vi "Simple Test Executive Test.vi"() -> ()   [LabVIEW 2017]
uses:
  <vilib>/gpm_packages/@cs/test-executive/Source/Test Executive/Executioner/Executioner.lvclass
  <vilib>/gpm_packages/@cs/persistence/source/XML/XML.lvclass
  C:/Program Files/National Instruments/LabVIEW 2017/vi.lib/gpm_packages/@cs/persistence/source/IPersist/IPersist.lvclass
  <vilib>/gpm_packages/@cs/test-executive/Source/Test Executive/TestExecutive/Test Executive.lvclass
  C:/Program Files/National Instruments/LabVIEW 2017/vi.lib/gpm_packages/@cs/test-executive/Source/Test Executive/ITestExecutive/ITest Executive.lvclass
  <vilib>/gpm_packages/@cs/run-time-assertions/Source/Assert Equal/Assert Equal.lvclass
  C:/Program Files/National Instruments/LabVIEW 2017/vi.lib/gpm_packages/@cs/run-time-assertions/Source/Assert/Assert.lvclass
  866dfd19-2fef-4b99-8a4a-1d31d88e504e.vi
  55b154ae-6d03-47ed-abc2-d28db7feda01.vi
  cb4faef1-3dab-41b9-9dd5-aad0424c17a6.vi
  bfcbba5b-45c6-4320-969f-3e3d3b66b4de.vi
  8564ab31-dd3a-4968-8861-3b4339f4920d.vi
  9b79477b-4d99-41b4-a2fb-9df7ea8afb31.vi
  6decda23-fb0c-4e77-ad71-e1f71655b843.vi
  71592cda-0d0e-4ea7-b138-086424aed341.vi
  0583369c-d912-4d49-be3f-0b23069dcf00.vi
  bffa5b7c-ecbc-40cd-a0d5-f9da2a76cf50.vi
  c9edba23-499d-4d6b-bf99-6c37c6a75b36.vi
  b25967a6-4fd7-4e76-b6fa-60230ccf68d8.vi
  5610abd5-5b24-4367-9a8b-cdb86ef1c489.vi
  b0752a74-c361-4210-a9fb-4ae4d881d9e9.vi
  8d04dc0f-32ed-4eef-804d-f0fb33ecb275.vi
  <vilib>/Utility/error.llb/Clear Errors.vi
  <vilib>/Utility/error.llb/Error Cluster From Error Code.vi
  <vilib>/gpm_packages/@cs/test-executive/Source/Test Executive/ITestExecutive/ITest Executive.lvclass
  <vilib>/gpm_packages/@cs/test-executive/Source/Test Executive/TestExecutive Ref/TestExecutive Ref.lvclass
panel:
  out "Attributes":i32[](array[numeric])
  out "Names":string[](array[string])
  out "Unique ID out":string
  out "Array":string[](array[string])
  out "Class":string
  out "Tag":i32
  out "Name":string
  out "Attribute 2":i32
  out "x = y?":bool
  out "variant":variant
  out "Attribute":variant
  out "class name":string
  in  "stop":bool
  out "error out":errorcluster
  in  "Loaded Test Exec":string(tree)
  out "Pointer?":bool
  in  "File Name":string
  in  "Folder":path
  in  "Saved Test Exec":string(tree)
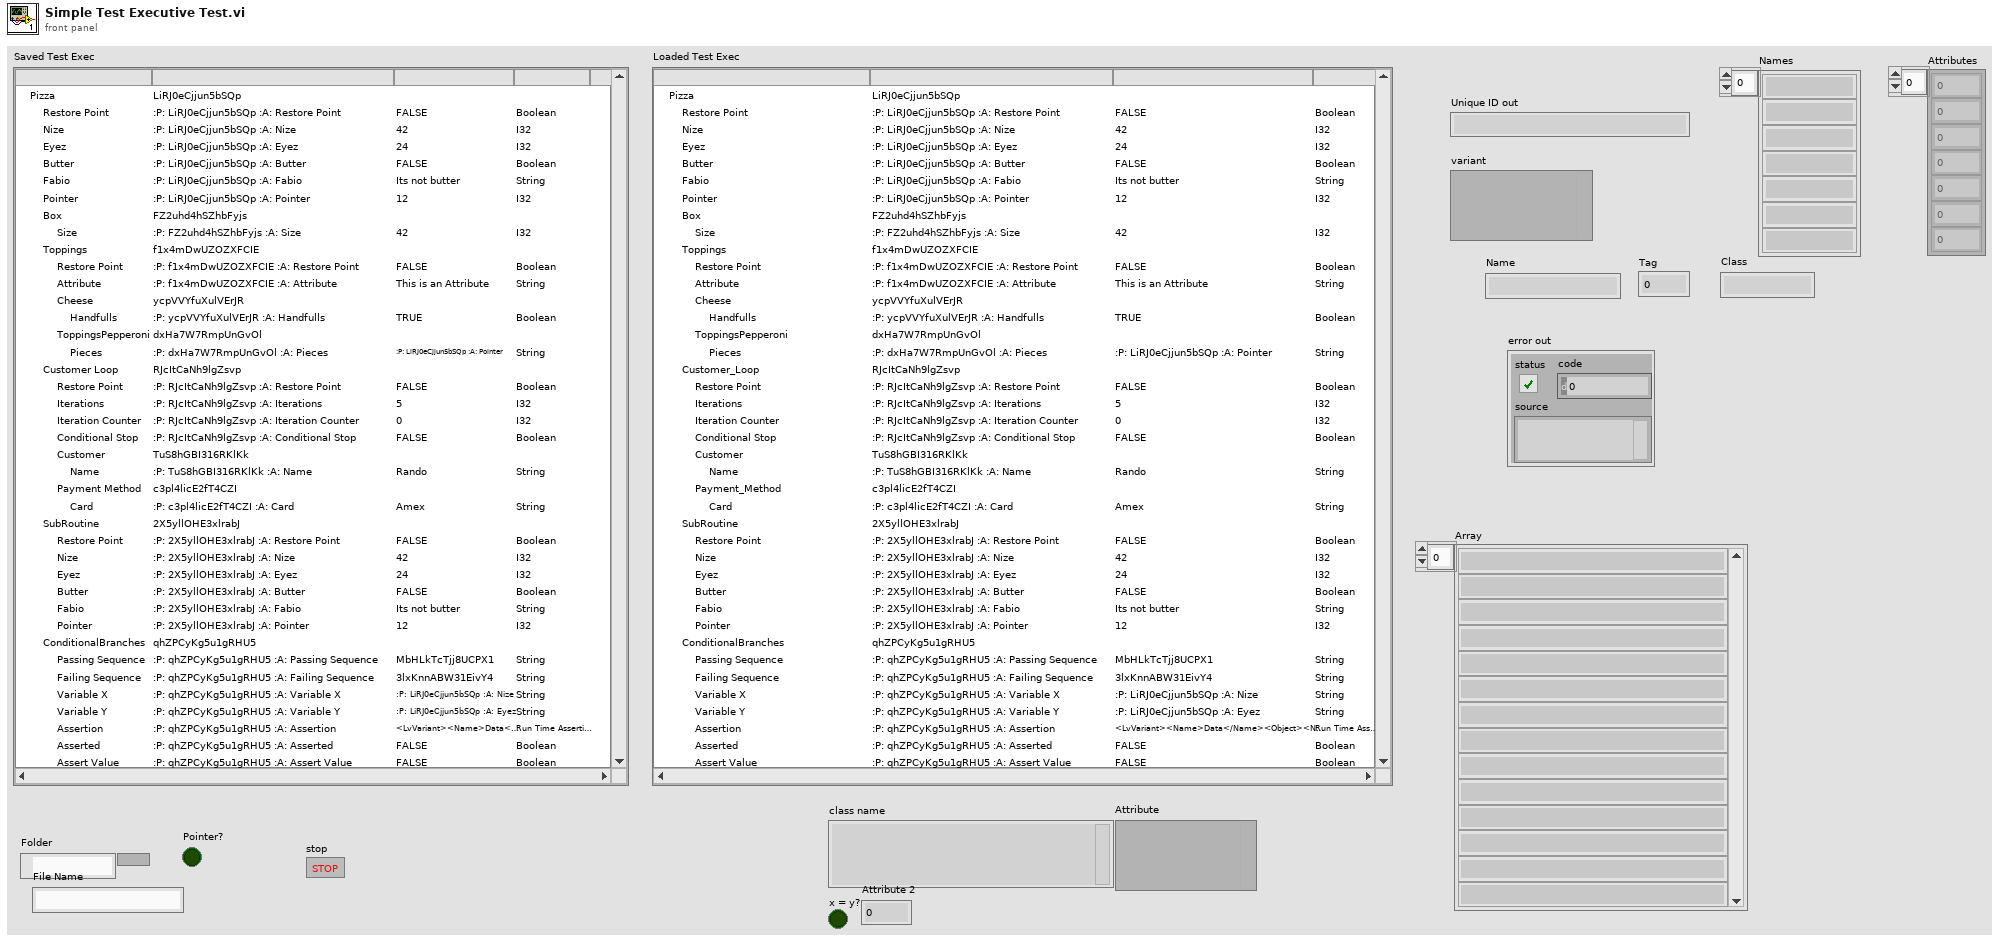
[diagram p1: front panel]
types:
  T1 = cluster{"Left Cell String":string, "Child Text":string[], "Child Tag":string, "Item Indent":i32, "Child Only?":bool, "Glyph Index":i32}[]
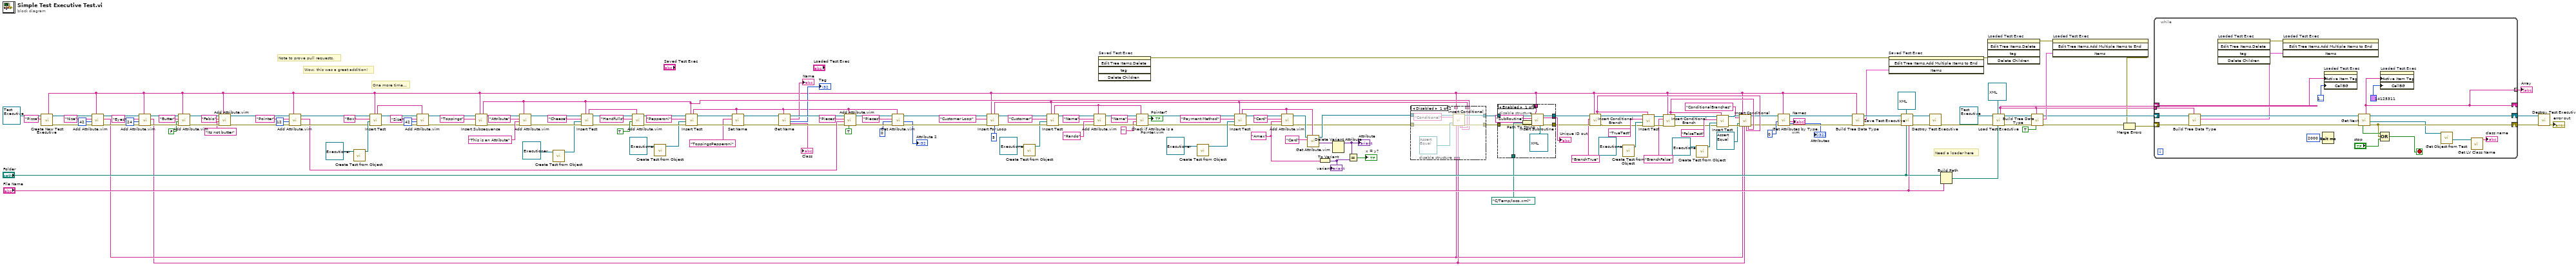
[diagram p0: block diagram]
diagram:
  w105 = "Amex"
  # "One more time..."
  # "Wow, this was a great addition!"
  # "Note to prove pull requests."
  # "Need a loader here"
  n1 = call <vilib>:"Create New Test Executive.vi"("Name"="Pizza", "Test Executive"=refnum<class "Test Executive.lvclass"> refnum ("Test Executive.lvlib:Test Executive.lvclass")) -> ("error out"=w99:errorcluster, "Test Executive Ref"=w100:refnum<data-value>, "Test Executive ID out"=w3:string)  [unwired: 7 in]
  n2 = call "Add Attribute.vim"("ID"=w3, "error in (no error)"=w99, "Attribute"=42, "Attribute Name"="Nize", "Test Executive Ref"=w100) -> ("error out"=w95:errorcluster, "Attribute ID out"=w5:string, "Test Executive Ref out"=w96:refnum<data-value>)  [unwired: 3 in, 1 out]
  n3 = call "Add Attribute.vim"("ID"=w3, "error in (no error)"=w95, "Attribute"=24, "Attribute Name"="Eyez", "Test Executive Ref"=w96) -> ("error out"=w36:errorcluster, "Attribute ID out"=w4:string, "Test Executive Ref out"=w37:refnum<data-value>)  [unwired: 3 in, 1 out]
  n4 = call "Add Attribute.vim"("ID"=w3, "error in (no error)"=w36, "Attribute"=FALSE, "Attribute Name"="Butter", "Test Executive Ref"=w37) -> ("error out"=w31:errorcluster, "Test Executive Ref out"=w33:refnum<data-value>)  [unwired: 3 in, 2 out]
  n5 = call "Add Attribute.vim"("ID"=w3, "error in (no error)"=w31, "Attribute"="Its not butter", "Attribute Name"="Fabio", "Test Executive Ref"=w33) -> ("error out"=w30:errorcluster, "Test Executive Ref out"=w32:refnum<data-value>)  [unwired: 3 in, 2 out]
  n6 = call "Add Attribute.vim"("ID"=w3, "error in (no error)"=w30, "Attribute"=12, "Attribute Name"="Pointer", "Test Executive Ref"=w32) -> ("error out"=w84:errorcluster, "Attribute ID out"=w82:string, "Test Executive Ref out"=w83:refnum<data-value>)  [unwired: 3 in, 1 out]
  n7 = call <vilib>:"Create Test from Object.vi"("Test"=refnum<class "Executioner.lvclass"> refnum ("Test Executive.lvlib:Executioner.lvclass")) -> ("Test"=w117:refnum<class "Executioner.lvclass">)  [unwired: 10 in]
  n8 = call <vilib>:"Insert Test.vi"("Parent ID"=w3, "error in (no error)"=w84, "Test"=w117, "Name"="Box", "Test Executive Ref"=w83) -> ("error out"=w141:errorcluster, "Test Executive Ref out"=w173:refnum<data-value>, "Unique ID out"=w172:string)  [unwired: 3 in, 1 out]
  n9 = call "Add Attribute.vim"("ID"=w172, "error in (no error)"=w141, "Attribute"=42, "Attribute Name"="Size", "Test Executive Ref"=w173) -> ("error out"=w91:errorcluster, "Test Executive Ref out"=w92:refnum<data-value>)  [unwired: 3 in, 2 out]
  n10 = call <vilib>:"Insert Subsequence.vi"("Parent ID"=w3, "error in (no error)"=w91, "Name"="Toppings", "Test Executive Ref"=w92) -> ("error out"=w140:errorcluster, "Test Executive Ref out"=w153:refnum<data-value>, "Unique ID out"=w87:string)  [unwired: 4 in, 1 out]
  n11 = call "Add Attribute.vim"("ID"=w87, "error in (no error)"=w140, "Attribute"="This is an Attribute", "Attribute Name"="Attribute", "Test Executive Ref"=w153) -> ("error out"=w139:errorcluster, "Test Executive Ref out"=w152:refnum<data-value>)  [unwired: 3 in, 2 out]
  n12 = call <vilib>:"Create Test from Object.vi"("Test"=refnum<class "Executioner.lvclass"> refnum ("Test Executive.lvlib:Executioner.lvclass")) -> ("Test"=w119:refnum<class "Executioner.lvclass">)  [unwired: 10 in]
  n13 = call <vilib>:"Insert Test.vi"("Parent ID"=w87, "error in (no error)"=w139, "Test"=w119, "Name"="Cheese", "Test Executive Ref"=w152) -> ("error out"=w138:errorcluster, "Test Executive Ref out"=w167:refnum<data-value>, "Unique ID out"=w166:string)  [unwired: 3 in, 1 out]
  n14 = call "Add Attribute.vim"("ID"=w166, "error in (no error)"=w138, "Attribute"=TRUE, "Attribute Name"="Handfulls", "Test Executive Ref"=w167) -> ("error out"=w137:errorcluster, "Test Executive Ref out"=w161:refnum<data-value>)  [unwired: 3 in, 2 out]
  n15 = call <vilib>:"Create Test from Object.vi"("Test"=refnum<class "Executioner.lvclass"> refnum ("Test Executive.lvlib:Executioner.lvclass")) -> ("Test"=w115:refnum<class "Executioner.lvclass">)  [unwired: 10 in]
  n16 = call <vilib>:"Insert Test.vi"("Parent ID"=w87, "error in (no error)"=w137, "Test"=w115, "Name"="Pepperoni", "Test Executive Ref"=w161) -> ("error out"=w66:errorcluster, "Test Executive Ref out"=w68:refnum<data-value>, "Unique ID out"=w64:string)  [unwired: 3 in, 1 out]
  n17 = call <vilib>:"Set Name.vi"("Unique ID"=w64, "error in (no error)"=w66, "Name"="ToppingsPepperoni", "Test Executive Ref"=w68) -> ("error out"=w65:errorcluster, "Test Executive Ref out"=w67:refnum<data-value>)  [unwired: 6 in]
  n18 = call <vilib>:"Get Name.vi"("Unique ID"=w64, "error in (no error)"=w65, "Test Executive Ref"=w67) -> ("error out"=w72:errorcluster, "Tag"=→"Tag":i32, "Name"=→"Name":string, "Test Executive Ref out"=w73:refnum<data-value>, "Class"=→"Class":string)  [unwired: 4 in]
  n19 = call "Add Attribute.vim"("Pointer?"=TRUE, "ID"=w64, "error in (no error)"=w72, "Attribute"=w82, "Attribute Name"="Pieces", "Test Executive Ref"=w73) -> ("error out"=w78:errorcluster, "Test Executive Ref out"=w80:refnum<data-value>)  [unwired: 2 in, 2 out]
  n20 = call "Get Attribute.vim"("ID"=w64, "error in (no error)"=w78, "Type"=0, "Attribute Name"="Pieces", "Test Executive Ref"=w80) -> ("error out"=w77:errorcluster, "Attribute"=→"Attribute 2":i32, "Test Executive Ref out"=w79:refnum<data-value>)  [unwired: 2 in, 2 out]
  n21 = call <vilib>:"Insert For Loop.vi"("Loop Iterations"=5, "Parent ID"=w3, "error in (no error)"=w77, "Name"="Customer Loop" ("Unique ID"), "Test Executive Ref"=w79) -> ("error out"=w128:errorcluster, "Test Executive Ref out"=w129:refnum<data-value>, "Unique ID out"=w88:string)  [unwired: 3 in, 1 out]
  n22 = call <vilib>:"Create Test from Object.vi"("Test"=refnum<class "Executioner.lvclass"> refnum ("Test Executive.lvlib:Executioner.lvclass")) -> ("Test"=w113:refnum<class "Executioner.lvclass">)  [unwired: 10 in]
  n23 = call <vilib>:"Insert Test.vi"("Parent ID"=w88, "error in (no error)"=w128, "Test"=w113, "Name"="Customer", "Test Executive Ref"=w129) -> ("error out"=w136:errorcluster, "Test Executive Ref out"=w158:refnum<data-value>, "Unique ID out"=w121:string)  [unwired: 3 in, 1 out]
  n24 = call "Add Attribute.vim"("ID"=w121, "error in (no error)"=w136, "Attribute"="Rando", "Attribute Name"="Name", "Test Executive Ref"=w158) -> ("error out"=w147:errorcluster, "Test Executive Ref out"=w148:refnum<data-value>)  [unwired: 3 in, 2 out]
  n25 = invoke on="Saved Test Exec" class="Tree (strict)" method="Edit Tree Items.Delete"() -> (error out=w156:errorcluster)  [unwired: 5 in, 4 out]
  n26 = call "Check if Attribute is a Pointer.vim"("ID"=w121, "error in (no error)"=w147, "Type"="", "Attribute Name"="Name", "Test Executive Ref"=w148) -> ("error out"=w93:errorcluster, "Pointer?"=→"Pointer?":bool, "Test Executive Ref out"=w94:refnum<data-value>)  [unwired: 2 in, 2 out]
  n27 = call <vilib>:"Create Test from Object.vi"("Test"=refnum<class "Executioner.lvclass"> refnum ("Test Executive.lvlib:Executioner.lvclass")) -> ("Test"=w111:refnum<class "Executioner.lvclass">)  [unwired: 10 in]
  n28 = call <vilib>:"Insert Test.vi"("Parent ID"=w88, "error in (no error)"=w93, "Test"=w111, "Name"="Payment Method", "Test Executive Ref"=w94) -> ("error out"=w125:errorcluster, "Test Executive Ref out"=w123:refnum<data-value>, "Unique ID out"=w109:string)  [unwired: 3 in, 1 out]
  n29 = call "Add Attribute.vim"("ID"=w109, "error in (no error)"=w125, "Attribute"=w105, "Attribute Name"="Card", "Test Executive Ref"=w123) -> ("error out"=w89:errorcluster, "Test Executive Ref out"=w110:refnum<data-value>)  [unwired: 3 in, 2 out]
  n30 = call "Get Attribute.vim"("ID"=w109, "Attribute Name"="Card", "Test Executive Ref"=w110) -> ("Attribute"=w104:variant, "Test Executive Ref out"=w90:refnum<data-value>)  [unwired: 4 in, 3 out]
  n31 = To Variant(anything=w105) -> (Variant=w107:variant)
  "variant" <- w107
  n32 = Delete Variant Attribute(7:w104) -> (3:w103:variant)  [unwired: 2 in, 2 out]
  "Attribute" <- w103
  n33 = Equal?(x=w103, y=w107) -> (x = y?=→"x = y?":bool)
  n34 = disable-structure shown="Disabled" {
    disable-tunnel: w5 -> [w185 _]
    disable-tunnel: w4 -> [w184 _]
    disable-tunnel: w90 -> [w183 w189]
    disable-tunnel: [w182 w189] -> w50
    disable-tunnel: w3 -> [w181 _]
    disable-tunnel: w89 -> [w180 w188]
    disable-tunnel: [w179 w188] -> w49
    disable-tunnel: w88 -> [w178 _]
    disable-tunnel: w87 -> [w177 _]
    frame Disabled {
      n35 = call <vilib>:"Insert Conditional.vi"("Test Executive Ref"=w183, "Name"="Conditional", "Assertion"=refnum<class "Assert Equal.lvclass"> refnum ("Run Time Assertions.lvlib:Assert Equal.lvclass"), "error in (no error)"=w180, "Parent ID"=w181, "Variable X"=w185, "Variable Y"=w184, "Passing Executive"=w178, "Failing Executive"=w177) -> ("Test Executive Ref out"=w182:refnum<data-value>, "error out"=w179:errorcluster)  [unwired: 7 in, 2 out]
    }
    frame Enabled {
    }
  }
  n36 = disable-structure shown="Enabled" {
    disable-tunnel: path "C:/Temp/loco.xml" -> [w197 _]
    disable-tunnel: [w196 _] -> w51
    disable-tunnel: w50 -> [w195 w201]
    disable-tunnel: w49 -> [w194 w200]
    disable-tunnel: [w193 w201] -> w27
    disable-tunnel: [w192 w200] -> w26
    disable-tunnel: w3 -> [w191 _]
    frame Enabled {
      n37 = Path To String(path=w197) -> (string=w190:string)
      n38 = call <vilib>:"Insert Subroutine.vi"("Test Executive Ref"=w195, "Parent ID"=w191, "Name"="SubRoutine", "Subroutine Path"=w190, "error in (no error)"=w194, "Persistence"=refnum<class "XML.lvclass"> refnum ("XML.lvlib:XML.lvclass")) -> ("Unique ID out"=w196:string, "Test Executive Ref out"=w193:refnum<data-value>, "error out"=w192:errorcluster)  [unwired: 6 in, 1 out]
    }
    frame Disabled {
    }
  }
  "Unique ID out" <- w51
  n39 = call <vilib>:"Insert Conditional Branch.vi"("Parent ID"=w3, "error in (no error)"=w26, "Name"="BranchTrue", "Test Executive Ref"=w27) -> ("error out"=w21:errorcluster, "Test Executive Ref out"=w20:refnum<data-value>, "Unique ID out"=w6:string)  [unwired: 4 in, 1 out]
  n40 = call <vilib>:"Create Test from Object.vi"("Test"=refnum<class "Executioner.lvclass"> refnum ("Test Executive.lvlib:Executioner.lvclass")) -> ("Test"=w22:refnum<class "Executioner.lvclass">)  [unwired: 10 in]
  n41 = call <vilib>:"Insert Test.vi"("Parent ID"=w6, "error in (no error)"=w21, "Test"=w22, "Name"="TrueTest", "Test Executive Ref"=w20) -> ("error out"=w14:errorcluster, "Test Executive Ref out"=w13:refnum<data-value>)  [unwired: 3 in, 2 out]
  n42 = call <vilib>:"Insert Conditional Branch.vi"("Parent ID"=w3, "error in (no error)"=w14, "Name"="BranchFalse", "Test Executive Ref"=w13) -> ("error out"=w16:errorcluster, "Test Executive Ref out"=w15:refnum<data-value>, "Unique ID out"=w7:string)  [unwired: 4 in, 1 out]
  n43 = call <vilib>:"Create Test from Object.vi"("Test"=refnum<class "Executioner.lvclass"> refnum ("Test Executive.lvlib:Executioner.lvclass")) -> ("Test"=w17:refnum<class "Executioner.lvclass">)  [unwired: 10 in]
  n44 = call <vilib>:"Insert Test.vi"("Parent ID"=w7, "error in (no error)"=w16, "Test"=w17, "Name"="FalseTest", "Test Executive Ref"=w15) -> ("error out"=w11:errorcluster, "Test Executive Ref out"=w10:refnum<data-value>)  [unwired: 3 in, 2 out]
  n45 = call <vilib>:"Insert Conditional.vi"("Test Executive Ref"=w10, "Name"="ConditionalBranches", "Assertion"=refnum<class "Assert Equal.lvclass"> refnum ("Run Time Assertions.lvlib:Assert Equal.lvclass"), "error in (no error)"=w11, "Parent ID"=w3, "Variable X"=w5, "Variable Y"=w4, "Passing Executive"=w6, "Failing Executive"=w7) -> ("Test Executive Ref out"=w1:refnum<data-value>, "error out"=w2:errorcluster)  [unwired: 7 in, 2 out]
  n46 = call "Get Attributes by Type.vim"("ID"=w3, "error in (no error)"=w2, "Type"=0, "Test Executive Ref"=w1) -> ("error out"=w41:errorcluster, "Names"=→"Names":string[], "Test Executive Ref out"=w42:refnum<data-value>, "Attributes"=→"Attributes":i32[])  [unwired: 3 in, 1 out]
  n47 = call <vilib>:"Build Tree Data Type.vi"("Test ID"=w3, "error in (no error)"=w41, "Test Executive Ref"=w42) -> ("error out"=w47:errorcluster, "Tree Data"=w46:T1, "Test Executive Ref out"=w48:refnum<data-value>)  [unwired: 6 in]
  n48 = invoke on="Saved Test Exec" class="Tree (strict)" method="Edit Tree Items.Add Multiple Items to End"(error in=w156, "Items"=w46) -> (error out=w45:errorcluster)  [unwired: 2 in, 3 out]
  n49 = call <vilib>:"Save Test Executive.vi"("File Name"="File Name", "Folder"="Folder", "Persistence in"=refnum<class "XML.lvclass"> refnum ("XML.lvlib:XML.lvclass"), "error in (no error)"=w47, "Test Executive Ref"=w48) -> ("error out"=w154:errorcluster, "Test Executive Ref out"=w155:refnum<data-value>)  [unwired: 5 in]
  n50 = call <vilib>:"Destroy Test Executive.vi"("error in (no error)"=w154, "Test Executive Ref"=w155) -> ("error out"=w133:errorcluster)  [unwired: 9 in]
  n51 = Build Path(base path="Folder", name or relative path="File Name") -> (appended path=w62:path)
  n52 = invoke on="Loaded Test Exec" class="Tree (strict)" method="Edit Tree Items.Delete"(error in=w45) -> (error out=w56:errorcluster)  [unwired: 4 in, 4 out]
  n53 = call <vilib>:"Load Test Executive.vi"("Folder"=w62, "Persistence in"=refnum<class "XML.lvclass"> refnum ("XML.lvlib:XML.lvclass"), "error in (no error)"=w133, "Test Executive"=refnum<class "Test Executive.lvclass"> refnum ("Test Executive.lvlib:Test Executive.lvclass")) -> ("error out"=w59:errorcluster, "Test Executive Ref out"=w60:refnum<data-value>, "Root ID"=w58:string)  [unwired: 5 in]
  n54 = call <vilib>:"Build Tree Data Type.vi"("Show IDs (True)"=TRUE, "Test ID"=w58, "error in (no error)"=w59, "Test Executive Ref"=w60) -> ("error out"=w53:errorcluster, "Tree Data"=w55:T1, "Test Executive Ref out"=w54:refnum<data-value>)  [unwired: 5 in]
  n55 = invoke on="Loaded Test Exec" class="Tree (strict)" method="Edit Tree Items.Add Multiple Items to End"(error in=w56, "Items"=w55) -> (error out=w43:errorcluster)  [unwired: 2 in, 3 out]
  n56 = Merge Errors(w53, w43) -> (w44:errorcluster)
  n57 = while {
    shift-right: [w221] -> w131
    shift-left: w54 -> [w209]
    shift-right: [w219] -> w130
    shift-left: w44 -> [w208]
    shift-right: [w202] -> _
    shift-left: w58 -> [w215]
    tunnel: w58 -> [w205]
    tunnel: [w202] -> w61 mode=indexing
    stop <- w217 stop-if-true
    n58 = call <vilib>:"Build Tree Data Type.vi"("Test ID"=w205, "error in (no error)"=w208, "Test Executive Ref"=w209) -> ("error out"=w207:errorcluster, "Tree Data"=w203:T1, "Test Executive Ref out"=w206:refnum<data-value>)  [unwired: 6 in]
    n59 = invoke on="Loaded Test Exec" class="Tree (strict)" method="Edit Tree Items.Delete"() -> (error out=w204:errorcluster)  [unwired: 5 in, 4 out]
    n60 = invoke on="Loaded Test Exec" class="Tree (strict)" method="Edit Tree Items.Add Multiple Items to End"(error in=w204, "Items"=w203) -> ()  [unwired: 2 in, 4 out]
    n61 = Wait (ms)(milliseconds to wait=u32 2000) -> ()  [unwired: 1 out]
    n62 = property on="Loaded Test Exec" class="Tree (strict)"("Active Item Tag"=w215, "CellBG"=u32 16777226) -> ()  [unwired: 2 in, 2 out]
    n63 = call <vilib>:"Get Next.vi"("error in (no error)"=w207, "Test Executive Ref"=w206) -> ("error out"=w219:errorcluster, "Test"=w212:refnum<class "Executioner.lvclass">, "Test Executive Ref out"=w221:refnum<data-value>, "Unique ID out"=w202:string, "Complete"=w220:bool)  [unwired: 3 in, 2 out]
    n64 = property on="Loaded Test Exec" class="Tree (strict)"("Active Item Tag"=w202, "CellBG"=u32 14125311) -> ()  [unwired: 2 in, 2 out]
    n65 = Compound Arithmetic op=OR(w220, w219, "stop") -> (w217:bool)
    n66 = call <vilib>:"Get Object from Test.vi"("Executioner in"=w212) -> ("Test"=w211:refnum<class>)  [unwired: 9 in, 1 out]
    n67 = call <vilib>:"Get LV Class Name.vi"("object"=w211) -> ("class name"=→"class name":string)  [unwired: 9 in, 1 out]
  }
  "Array" <- w61
  n68 = call <vilib>:"Destroy Test Executive.vi"("error in (no error)"=w130, "Test Executive Ref"=w131) -> ("error out"=→"error out":errorcluster)  [unwired: 9 in]
